vi "GetAllAlarmStatus.vi"(8 "error in":errorcluster, 11 "VISA resource name":refnum<visa-resource-name>) -> (0 "error out":errorcluster, 3 "VISA resource name out":refnum<visa-resource-name>)   [LabVIEW 2023, in "Thermotron 8800.lvlib"]
uses:
  Thermotron 8800.lvlib
  Private/AnalogInputChannelNumber 1-4.ctl
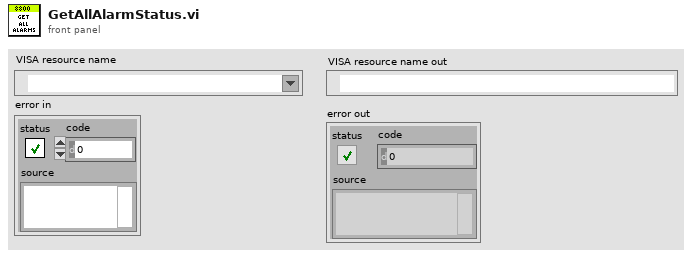
[diagram p1: front panel]
types:
  T1 = typedef "Thermotron 8800.lvlib/AnalogInputChannelNumber 1-4.ctl" = u16
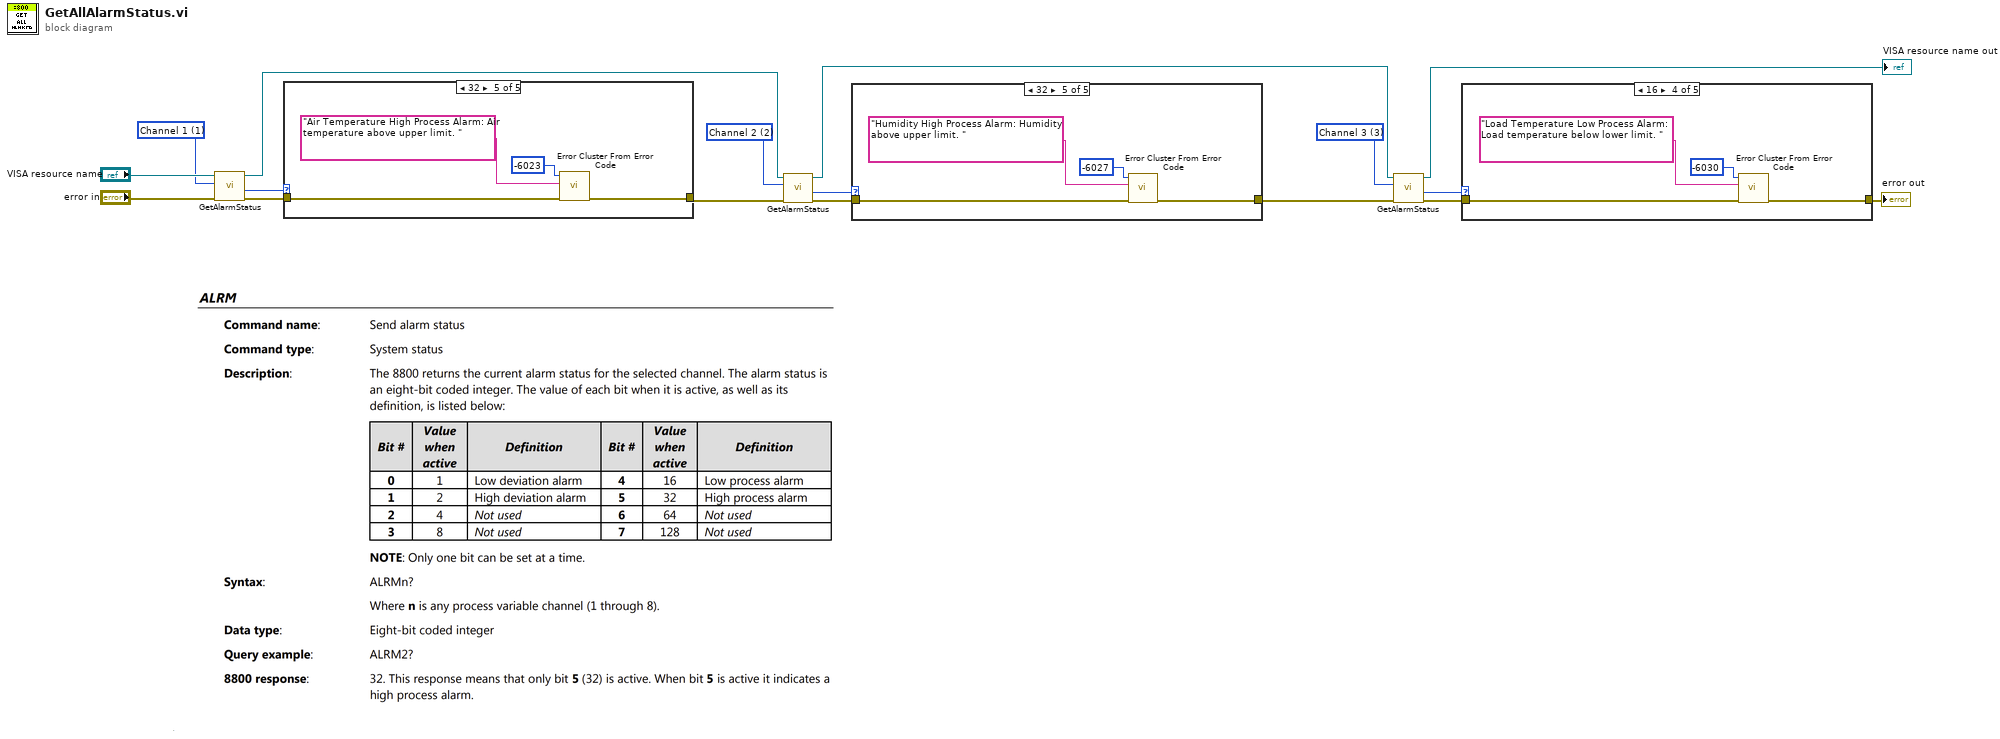
[diagram p0: block diagram]
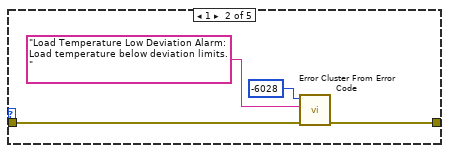
[diagram p3: hidden frame]
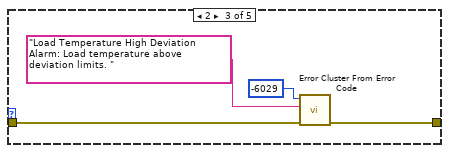
[diagram p4: hidden frame]
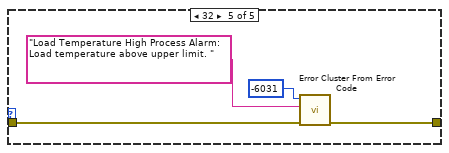
[diagram p5: hidden frame]
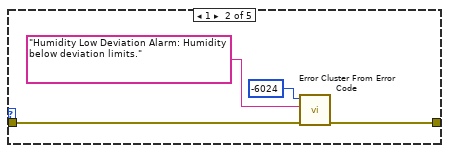
[diagram p7: hidden frame]
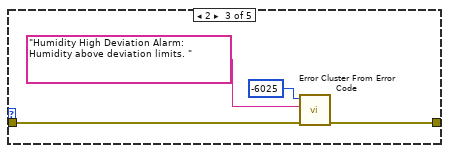
[diagram p8: hidden frame]
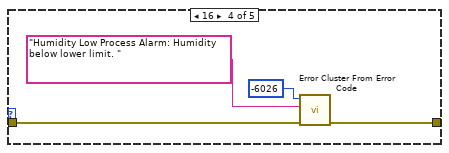
[diagram p9: hidden frame]
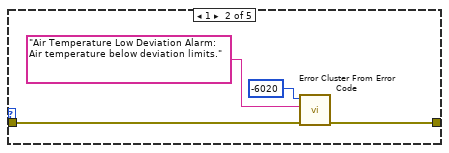
[diagram p11: hidden frame]
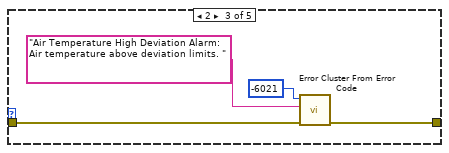
[diagram p12: hidden frame]
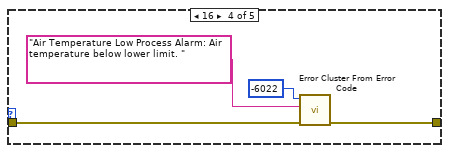
[diagram p13: hidden frame]
diagram:
  w7 = T1 3 items=["Channel 1"=1, "Channel 2"=2, "Channel 3"=3, "Channel 4"=4, "Channel 5"=5, "Channel 6"=6, "Channel 7"=7, "Channel 8"=8] ("Channel Number")
  w10 = T1 2 items=["Channel 1"=1, "Channel 2"=2, "Channel 3"=3, "Channel 4"=4, "Channel 5"=5, "Channel 6"=6, "Channel 7"=7, "Channel 8"=8] ("Channel Number")
  w15 = T1 1 items=["Channel 1"=1, "Channel 2"=2, "Channel 3"=3, "Channel 4"=4, "Channel 5"=5, "Channel 6"=6, "Channel 7"=7, "Channel 8"=8] ("Channel Number")
  n1 = call "GetAlarmStatus.vi"("error in"="error in", "Channel Number"=w15, "VISA resource name"="VISA resource name") -> ("error out"=w13:errorcluster, "Alarm status"=w14:i32, "VISA resource name out"=w8:refnum<visa-resource-name>)  [unwired: 5 in, 1 out]
  n2 = case shown="32" w14 {
    tunnel: w13 -> [w18 w22 w26 w30 w34]
    tunnel: [w18 w19 w23 w27 w31] -> w9
    frame 0, Default {
    }
    frame 1 {
      n3 = call <vilib>:"Error Cluster From Error Code.vi"("error in (no error)"=w22, "error message (\"\")"="Air Temperature Low Deviation Alarm: Air temperature below deviation limits." ("error message (\"\")"), "error code (0)"=-6020) -> ("error out"=w19:errorcluster)  [unwired: 6 in]
    }
    frame 2 {
      n4 = call <vilib>:"Error Cluster From Error Code.vi"("error in (no error)"=w26, "error message (\"\")"="Air Temperature High Deviation Alarm: Air temperature above deviation limits. " ("error message (\"\")"), "error code (0)"=-6021) -> ("error out"=w23:errorcluster)  [unwired: 6 in]
    }
    frame 16 {
      n5 = call <vilib>:"Error Cluster From Error Code.vi"("error in (no error)"=w30, "error message (\"\")"="Air Temperature Low Process Alarm: Air temperature below lower limit. " ("error message (\"\")"), "error code (0)"=-6022) -> ("error out"=w27:errorcluster)  [unwired: 6 in]
    }
    frame 32 {
      n6 = call <vilib>:"Error Cluster From Error Code.vi"("error in (no error)"=w34, "error message (\"\")"="Air Temperature High Process Alarm: Air temperature above upper limit. " ("error message (\"\")"), "error code (0)"=-6023) -> ("error out"=w31:errorcluster)  [unwired: 6 in]
    }
  }
  n7 = call "GetAlarmStatus.vi"("error in"=w9, "Channel Number"=w10, "VISA resource name"=w8) -> ("error out"=w12:errorcluster, "Alarm status"=w11:i32, "VISA resource name out"=w3:refnum<visa-resource-name>)  [unwired: 5 in, 1 out]
  n8 = case shown="32" w11 {
    tunnel: w12 -> [w35 w39 w43 w47 w51]
    tunnel: [w35 w36 w40 w44 w48] -> w4
    frame 0, Default {
    }
    frame 1 {
      n9 = call <vilib>:"Error Cluster From Error Code.vi"("error in (no error)"=w39, "error message (\"\")"="Humidity Low Deviation Alarm: Humidity below deviation limits." ("error message (\"\")"), "error code (0)"=-6024) -> ("error out"=w36:errorcluster)  [unwired: 6 in]
    }
    frame 2 {
      n10 = call <vilib>:"Error Cluster From Error Code.vi"("error in (no error)"=w43, "error message (\"\")"="Humidity High Deviation Alarm: Humidity above deviation limits. " ("error message (\"\")"), "error code (0)"=-6025) -> ("error out"=w40:errorcluster)  [unwired: 6 in]
    }
    frame 16 {
      n11 = call <vilib>:"Error Cluster From Error Code.vi"("error in (no error)"=w47, "error message (\"\")"="Humidity Low Process Alarm: Humidity below lower limit. " ("error message (\"\")"), "error code (0)"=-6026) -> ("error out"=w44:errorcluster)  [unwired: 6 in]
    }
    frame 32 {
      n12 = call <vilib>:"Error Cluster From Error Code.vi"("error in (no error)"=w51, "error message (\"\")"="Humidity High Process Alarm: Humidity above upper limit. " ("error message (\"\")"), "error code (0)"=-6027) -> ("error out"=w48:errorcluster)  [unwired: 6 in]
    }
  }
  n13 = call "GetAlarmStatus.vi"("error in"=w4, "Channel Number"=w7, "VISA resource name"=w3) -> ("error out"=w5:errorcluster, "Alarm status"=w6:i32, "VISA resource name out"=→"VISA resource name out":refnum<visa-resource-name>)  [unwired: 5 in, 1 out]
  n14 = case shown="16" w6 {
    tunnel: w5 -> [w52 w56 w60 w64 w68]
    tunnel: [w52 w53 w57 w61 w65] -> w2
    frame 0, Default {
    }
    frame 1 {
      n15 = call <vilib>:"Error Cluster From Error Code.vi"("error in (no error)"=w56, "error message (\"\")"="Load Temperature Low Deviation Alarm: Load temperature below deviation limits." ("error message (\"\")"), "error code (0)"=-6028) -> ("error out"=w53:errorcluster)  [unwired: 6 in]
    }
    frame 2 {
      n16 = call <vilib>:"Error Cluster From Error Code.vi"("error in (no error)"=w60, "error message (\"\")"="Load Temperature High Deviation Alarm: Load temperature above deviation limits. " ("error message (\"\")"), "error code (0)"=-6029) -> ("error out"=w57:errorcluster)  [unwired: 6 in]
    }
    frame 16 {
      n17 = call <vilib>:"Error Cluster From Error Code.vi"("error in (no error)"=w64, "error message (\"\")"="Load Temperature Low Process Alarm: Load temperature below lower limit. " ("error message (\"\")"), "error code (0)"=-6030) -> ("error out"=w61:errorcluster)  [unwired: 6 in]
    }
    frame 32 {
      n18 = call <vilib>:"Error Cluster From Error Code.vi"("error in (no error)"=w68, "error message (\"\")"="Load Temperature High Process Alarm: Load temperature above upper limit. " ("error message (\"\")"), "error code (0)"=-6031) -> ("error out"=w65:errorcluster)  [unwired: 6 in]
    }
  }
  "error out" <- w2
